vi "HP34401A.vi"(4 "error in":T14, 7 "Command":T15) -> (0 "error out":T14, 3 "Response":T12)   [LabVIEW 2018]
uses:
  MOKO_LabViewLibrary/MokoLowLevel/MokoLowLovelControl/MLLC_Command.ctl
  MOKO_LabViewLibrary/MokoLowLevel/MokoLowLovelControl/MLLC_Error.ctl
  MOKO_LabViewLibrary/MokoLowLevel/MokoLowLovelControl/MLLC_Mode.ctl
  MOKO_LabViewLibrary/MokoLowLevel/MokoLowLovelControl/MLLC_Response.ctl
  MOKO_LabViewLibrary/MokoLowLevel/MokoLowLovelControl/MLLC_DriverName.ctl
  MOKO_LabViewLibrary/MokoLowLevel/MokoLowLovelControl/MLLC_Request.ctl
  MOKO_LabViewLibrary/MokoLowLevel/MokoLowLovelControl/MLLC_ErrorCode.ctl
  MOKO_LabViewLibrary/MokoLowLevel/MokoLowLovelControl/MLLC_ResponseInit.ctl
  MOKO_LabViewLibrary/MokoLowLevel/MokoLowLovelControl/MLLC_ConnectCluster.ctl
  MOKO_LabViewLibrary/MokoLowLevel/MokoLowLovelControl/MLLC_InterfaceType.ctl
  MOKO_LabViewLibrary/MokoLowLevel/MokoLowLovelControl/MLLC_OpenedSession.ctl
  MOKO_LabViewLibrary/MokoLowLevel/MokoLowLovelControl/MLLC_InterfaceSettings.ctl
  MOKO_LabViewLibrary/MokoLowLevel/MokoLowLovelControl/MLLC_InterfaceKind.ctl
  data/HP34401A_Functions.ctl
  MOKO_LabViewLibrary/MokoLowLevel/MokoLowLovelControl/MLLC_Delay.ctl
panel:
  in  "Settings":T8={"Saved Data"=variant, "Data"={"Connect"={"InterfaceType"=enum."VISA", "OpenedSession"="", "InterfaceSettings"={"Interface"=enum."RS232", "EOS 4 read"=enum."LF (\\n)", "EOS 4 write"=enum."CR+LF (\\r\\n)", "TMO, ms"=5000, "Sett"=variant(cluster{"Baud Rate":u32, "Data Bits":u16, "Parity":u16, "Stop Bits":u16, "Flow Control":u16, "Eho":bool} {"Baud Rate"=75, "Data Bits"=0, "Parity"=0, "Stop Bits"=0, "Flow Control"=0, "Eho"=FALSE})}}, "Channel"=1, "Func"=enum."VDC"}}
  in  "Response Init array":T9="HEWLETT-PACKARD,34401A,0,10-5-2"
  in  "Error Code":T6=5475
  in  "Request":T10="*idn?"
  in  "Driver Name":T11="HP34401A_GERMAN"
  in  "Mode":T13=enum."Check"
  # "HP34401A"
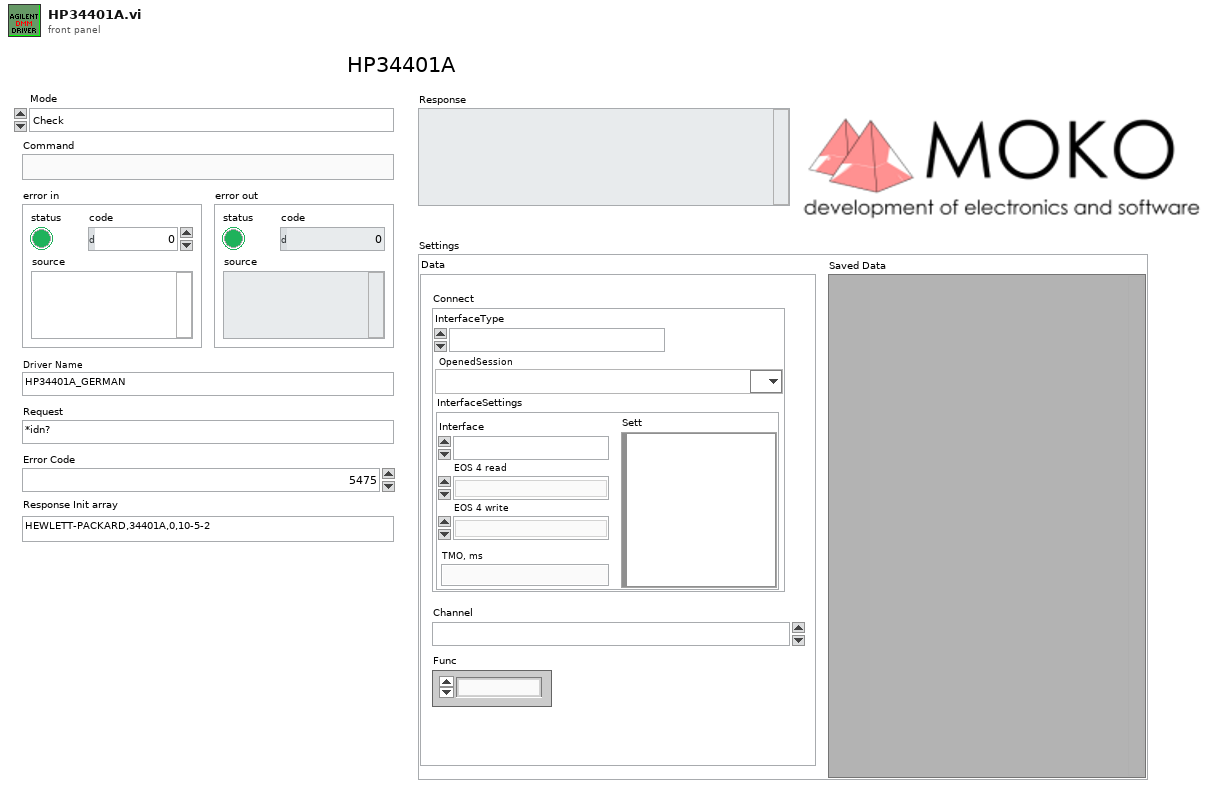
[diagram p1: front panel]
types:
  T1 = typedef "MLLC_ConnectCluster.ctl" = cluster{"InterfaceType":T2, "OpenedSession":T3, "InterfaceSettings":T4}
  T2 = typedef "MLLC_InterfaceType.ctl" = enum16{"VISA", "Prologix USB-GPIB"}
  T3 = typedef "MLLC_OpenedSession.ctl" = refnum<visa-resource-name>
  T4 = typedef "MLLC_InterfaceSettings.ctl" = cluster{"Interface":T5, "EOS 4 read":enum16{"Default (=EOS 4 write)", "CR (\\r)", "LF (\\n)", "None"}, "EOS 4 write":enum16{"CR+LF (\\r\\n)", "CR (\\r)", "LF (\\n)", "None"}, "TMO, ms":i32, "Sett":variant}
  T5 = typedef "MLLC_InterfaceKind.ctl" = enum16{"RS232", "GPIB", "USB", "Ethernet", "another"}
  T6 = typedef "MLLC_ErrorCode.ctl" = u32
  T7 = typedef "HP34401A_Functions.ctl" = enum16{"VDC", "VAC", "IDC", "IAC", "F", "R2", "R4", "CAP"}
  T8 = cluster{"Saved Data":variant, "Data":cluster{"Connect":T1, "Channel":T6, "Func":T7}}
  T9 = typedef "MLLC_ResponseInit.ctl" = string
  T10 = typedef "MLLC_Request.ctl" = string
  T11 = typedef "MLLC_DriverName.ctl" = string
  T12 = typedef "MLLC_Response.ctl" = string
  T13 = typedef "MLLC_Mode.ctl" = enum16{"get", "set", "close", "Init", "Check"}
  T14 = typedef "MLLC_Error.ctl" = errorcluster
  T15 = typedef "MLLC_Command.ctl" = string
  T16 = typedef "MLLC_Delay.ctl" = dbl
  T17 = typedef "MLLC_ResponseInitArray.ctl" = T9[]
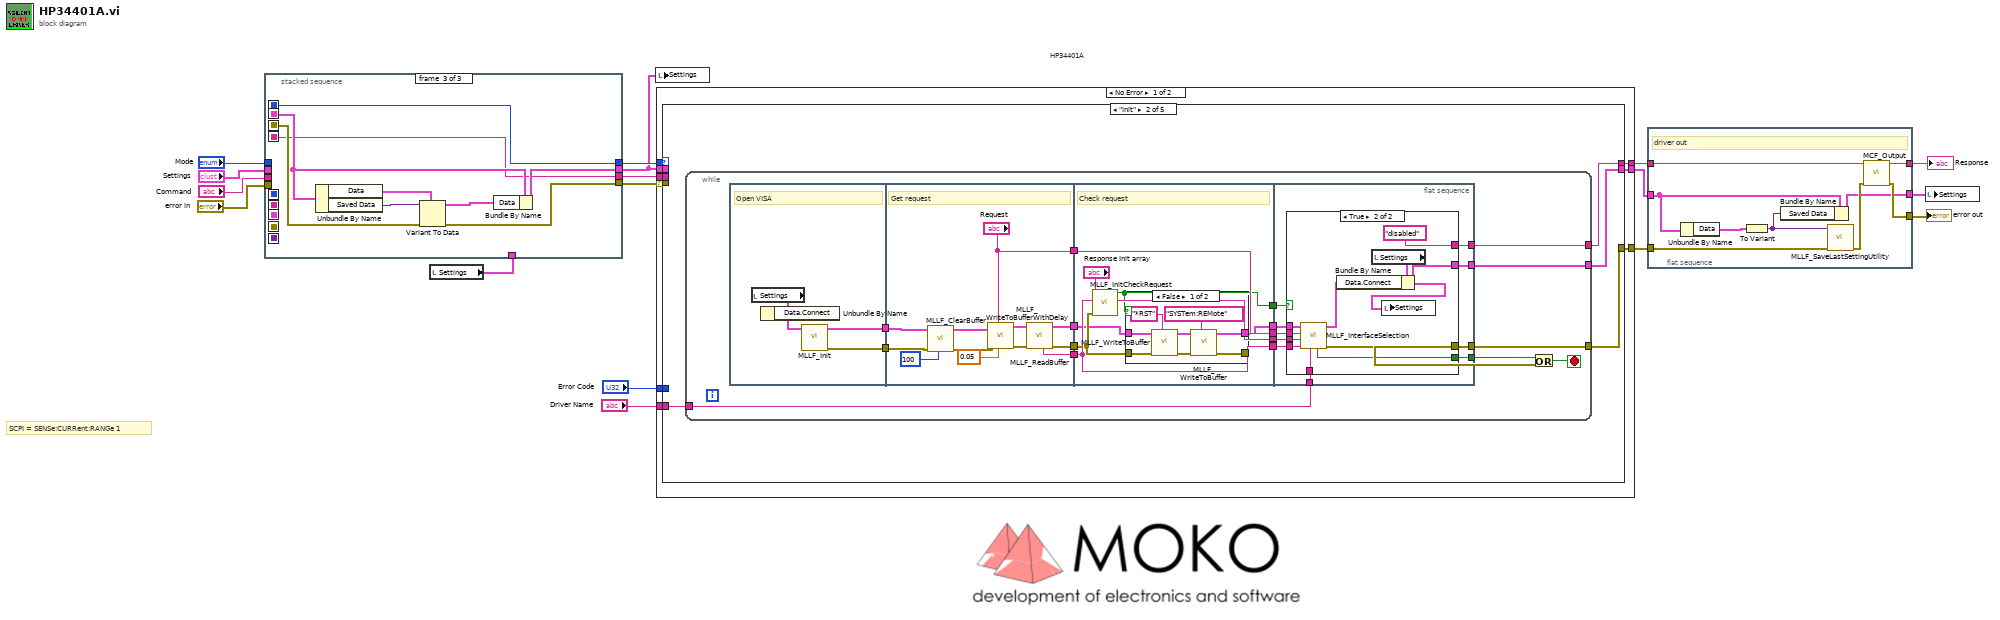
[diagram p0: block diagram]
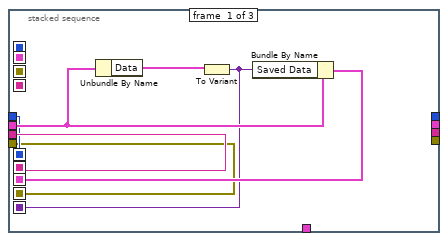
[diagram p2: hidden frame]
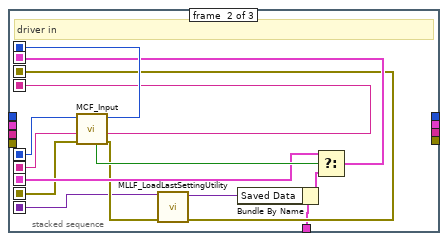
[diagram p3: hidden frame]
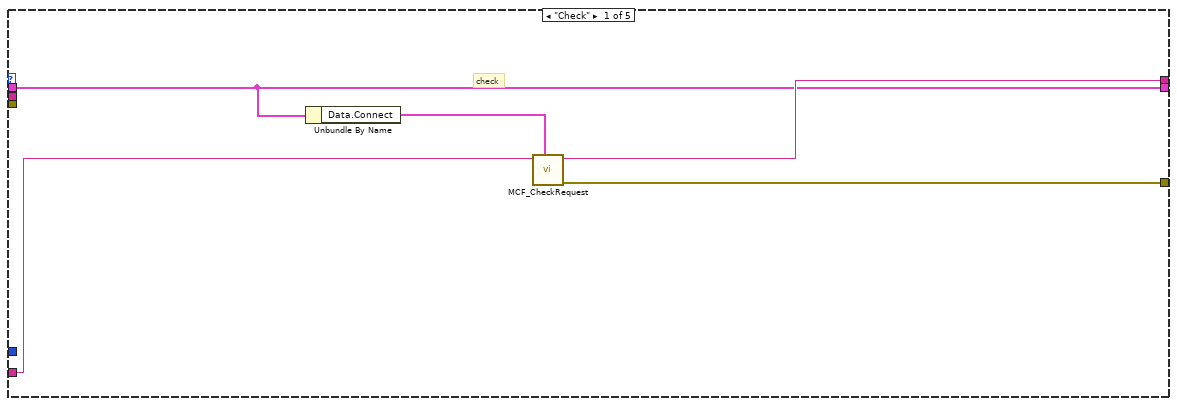
[diagram p4: hidden frame]
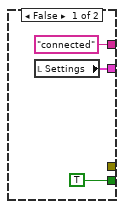
[diagram p6: hidden frame]
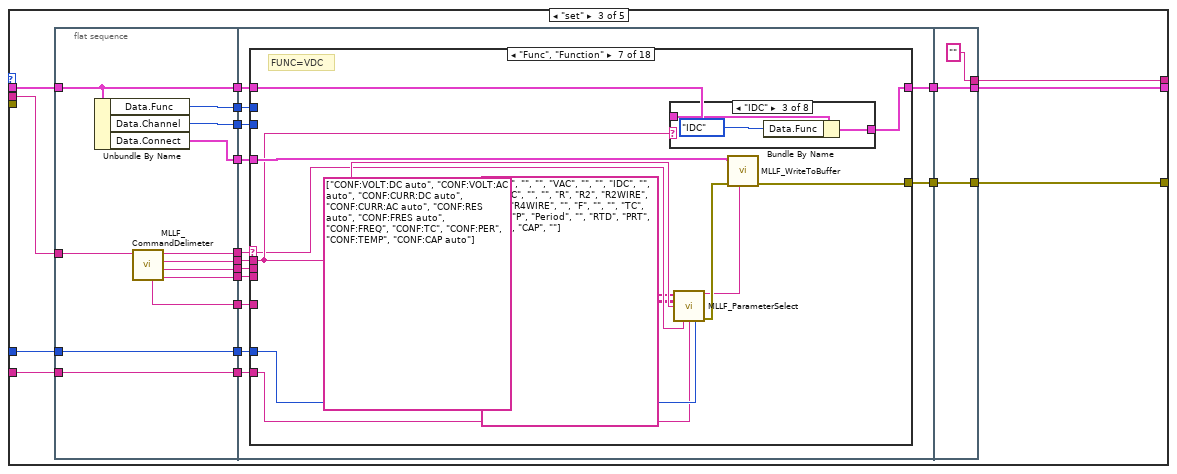
[diagram p7: hidden frame]
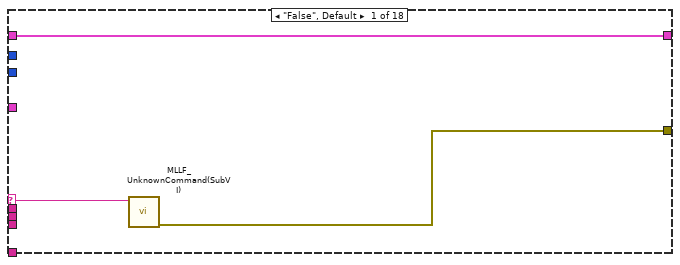
[diagram p8: hidden frame]
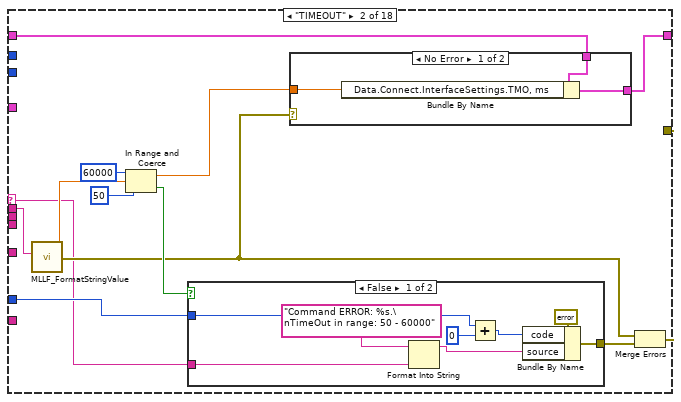
[diagram p9: hidden frame]
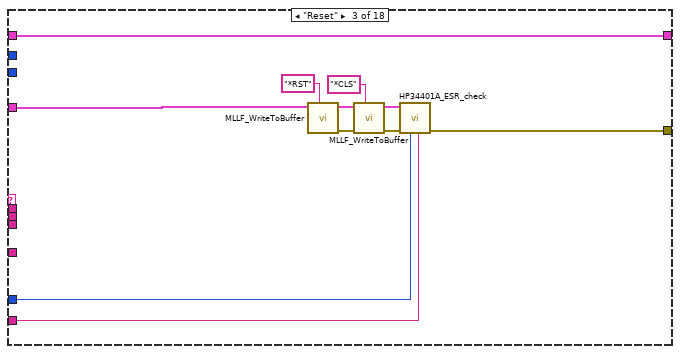
[diagram p12: hidden frame]
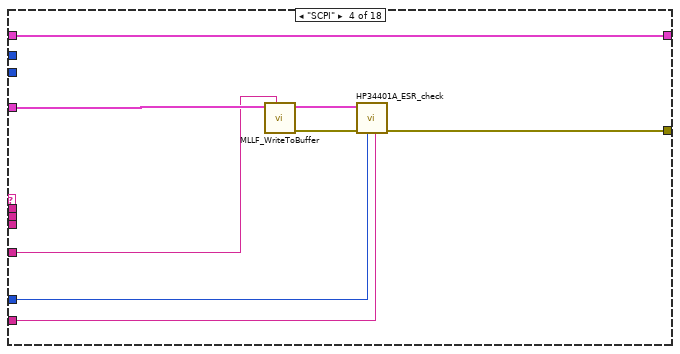
[diagram p13: hidden frame]
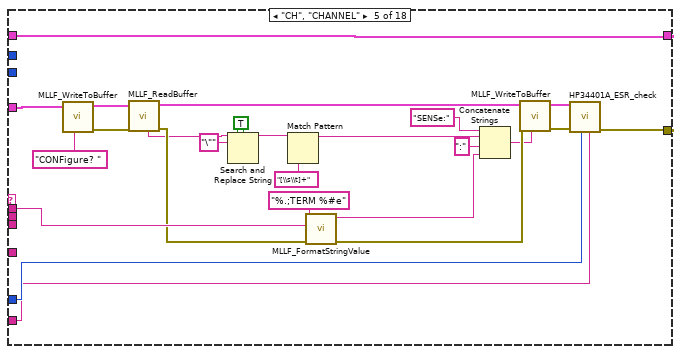
[diagram p14: hidden frame]
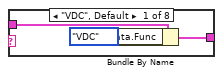
[diagram p16: hidden frame]
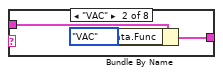
[diagram p17: hidden frame]
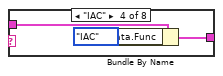
[diagram p18: hidden frame]
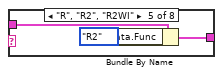
[diagram p19: hidden frame]
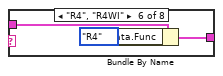
[diagram p20: hidden frame]
diagram:
  # "SCPI = SENSe:CURRent:RANGe 1"
  # "HP34401A"
  n1 = local read "Settings"() -> (w8:T8)
  n2 = stacked-sequence {
    seq-local: [w20 _ _] -> [_ w36 _]
    seq-local: [w19 _ _] -> [_ w37 _]
    seq-local: [w22 _ _] -> [_ w32 _]
    seq-local: [w18 _ _] -> [_ w31 _]
    seq-local: [w21 _ _] -> [_ w27 _]
    seq-local: [_ w28 _] -> [_ _ w44]
    seq-local: [_ w38 _] -> [_ _ w41]
    seq-local: [_ w35 _] -> [_ _ w40]
    seq-local: [_ w34 _] -> [_ _ w45]
    tunnel: "Command" -> [w20 _ _]
    tunnel: "Mode" -> [w19 _ _]
    tunnel: "error in" -> [w18 _ _]
    tunnel: "Settings" -> [w23 _ _]
    tunnel: w8 -> [_ w26 _]
    tunnel: [_ _ w40] -> w10
    tunnel: [_ _ w43] -> w1
    tunnel: [_ _ w42] -> w9
    tunnel: [_ _ w41] -> w11
    frame #0 {
      n3 = Unbundle By Name(w23) -> ("Data"=w24:cluster{"Connect":T1, "Channel":T6, "Func":T7})
      n4 = To Variant(anything=w24) -> (Variant=w21:variant)
      n5 = Bundle By Name(cluster=w23, "Saved Data"=w21) -> (w22:T8)
    }
    frame #1 {
      # "driver in"
      n6 = call "MCF_Input.vi"("Error In"=w31, "Command in"=w36, "Mode in"=w37) -> ("Error Out"=w30:errorcluster, "Command out"=w35:string, "Mode out"=w38:T13, "Boolean"=w33:bool)  [unwired: 5 in]
      n7 = call "MLLF_LoadLastSettingUtility.vi"("Error In"=w30, "Save data in"=w27) -> ("Error Out"=w28:errorcluster, "Save data out"=w25:variant)  [unwired: 8 in]
      n8 = Bundle By Name(cluster=w26, "Saved Data"=w25) -> (w29:T8)
      n9 = Select(t=w32, s=w33, f=w29) -> (s? t:f=w34:T8)
    }
    frame #2 {
      n10 = Unbundle By Name(w45) -> ("Data"=w46:cluster{"Connect":T1, "Channel":T6, "Func":T7}, "Saved Data"=w39:variant)
      n11 = Variant To Data(error in=w44, type=w46, Variant=w39) -> (data=w47:cluster{"Connect":T1, "Channel":T6, "Func":T7}, error out=w42:errorcluster)
      n12 = Bundle By Name(cluster=w45, "Data"=w47) -> (w43:T8)
    }
  }
  n13 = local write "Settings"(w1) -> ()
  n14 = case shown="No Error" w9 {
    selector: w9 -> [w53 w658]
    tunnel: [w54 w658] -> w5
    tunnel: w11 -> [w56 _]
    tunnel: [w55 "An error occurred in the driver input module." ("String")] -> w7
    tunnel: w10 -> [w48 _]
    tunnel: w1 -> [w49 w657]
    tunnel: "Error Code" -> [w52 _]
    tunnel: "Driver Name" -> [w51 _]
    tunnel: [w50 w657] -> w6
    frame No Error {
      n15 = case shown="\"Init\"" w56 {
        tunnel: [w60 w65 w153 w572 "" ("String")] -> w55
        tunnel: [w61 w63 w156 w573 w654] -> w54
        tunnel: w53 -> [_ _ _ w587 _]
        tunnel: w52 -> [_ _ w159 w589 _]
        tunnel: w51 -> [w59 w62 w157 w588 _]
        tunnel: [w57 w64 w158 w590 w653] -> w50
        tunnel: w49 -> [w57 _ w142 w578 w653]
        tunnel: w48 -> [_ _ w141 w577 _]
        frame "Check" {
          # "check"
          n16 = Unbundle By Name(w57) -> ("Data.Connect"=w58:T1)
          n17 = call "MCF_CheckRequest.vi"("Permanent data.Connect"=w58, "Driver Name"=w59) -> ("Error Out"=w61:errorcluster, "Output String"=w60:string)  [unwired: 8 in]
        }
        frame "Init" {
          n18 = while {
            tunnel: [w71] -> w63
            tunnel: [w70] -> w65
            tunnel: [w69] -> w64
            tunnel: w62 -> [w73]
            stop <- w82 stop-if-true
            n19 = flat-sequence {
              tunnel: [w86] -> w81
              tunnel: [w85] -> w80
              tunnel: w81 -> [w90]
              tunnel: w80 -> [w91]
              tunnel: [w96] -> w79
              tunnel: [w95] -> w78
              tunnel: [w94] -> w77
              tunnel: ["Request"] -> w67
              tunnel: w79 -> [w101]
              tunnel: w78 -> [w100]
              tunnel: w77 -> [w106]
              tunnel: [w99] -> w76
              tunnel: [w106] -> w75
              tunnel: [w102] -> w74
              tunnel: [w104] -> w68
              tunnel: w67 -> [w103]
              tunnel: [w103] -> w66
              tunnel: w76 -> [w124]
              tunnel: w75 -> [w123]
              tunnel: w74 -> [w125]
              tunnel: w73 -> [w122]
              tunnel: [w121] -> w72
              tunnel: [w120] -> w71
              tunnel: [w119] -> w70
              tunnel: [w118] -> w69
              tunnel: w68 -> [w117]
              tunnel: w66 -> [w116]
              frame #0 {
                # "Open VISA"
                n20 = local read "Settings"() -> (w84:T8)
                n21 = Unbundle By Name(w84) -> ("Data.Connect"=w83:T1)
                n22 = call "MLLF_Init.vi"("DriverConnect in"=w83) -> ("Error Out"=w86:errorcluster, "DriverConnect out"=w85:T1)  [unwired: 7 in]
              }
              frame #1 {
                # "Get request"
                n23 = call "MLLF_ClearBuffer.vi"("Timeout(default = 300 ms)"=u32 100, "Error In"=w90, "DriverConnect in"=w91) -> ("Error Out"=w88:errorcluster, "DriverConnect out"=w89:T1)  [unwired: 5 in, 1 out]
                n24 = call "MLLF_WriteToBufferWithDelay.vi"("Delay Time ( 0,05 s)"=T16 0.05, "Command"="Request", "Error In"=w88, "DriverConnect in"=w89) -> ("Error Out"=w97:errorcluster, "DriverConnect out"=w98:T1)  [unwired: 6 in]
                n25 = call "MLLF_ReadBuffer.vi"("Error In"=w97, "DriverConnect in"=w98) -> ("Error Out"=w96:errorcluster, "DriverConnect out"=w95:T1, "String"=w94:string)  [unwired: 6 in]
              }
              frame #2 {
                # "Check request"
                n26 = call "MLLF_InitCheckRequest.vi"("error in (no error)"=w101, "Answer"=w106, "Response Init"="Response Init array") -> ("ResponseInit out"=w104:string, "Design"=w102:bool)  [unwired: 5 in, 2 out]
                n27 = case shown="False" w102 {
                  tunnel: w101 -> [w110 _]
                  tunnel: w100 -> [w109 w115]
                  tunnel: [w108 w115] -> w99
                  tunnel: [w107 _] -> _
                  frame False {
                    n28 = call "MLLF_WriteToBuffer.vi"("String"="*RST", "error in"=w110, "DriverConnect in"=w109) -> ("error out"=w111:T14, "DriverConnect out"=w112:T1)  [unwired: 5 in]
                    n29 = call "MLLF_WriteToBuffer.vi"("String"="SYSTem:REMote", "error in"=w111, "DriverConnect in"=w112) -> ("error out"=w107:T14, "DriverConnect out"=w108:T1)  [unwired: 5 in]
                  }
                  frame True {
                  }
                }
              }
              frame #3 {
                n30 = case shown="True" w125 {
                  tunnel: w124 -> [_ w138]
                  tunnel: [TRUE w133] -> w121
                  tunnel: [_ w136] -> w120
                  tunnel: ["connected" "disabled"] -> w119
                  tunnel: [w126 w134] -> w118
                  tunnel: w123 -> [_ w131]
                  tunnel: w122 -> [_ w132]
                  tunnel: w117 -> [_ w130]
                  tunnel: w116 -> [_ w129]
                  frame False {
                    n31 = local read "Settings"() -> (w126:T8)
                  }
                  frame True {
                    n32 = call "MLLF_InterfaceSelection.vi"("Driver Name"=w132, "Answer:"=w131, "Response"=w130, "Request"=w129, "DriverConnect in"=w138) -> ("error out"=w136:T14, "DriverConnect out"=w137:T1, "stop init?"=w133:bool)  [unwired: 2 in, 2 out]
                    n33 = local read "Settings"() -> (w139:T8)
                    n34 = Bundle By Name(cluster=w139, "Data.Connect"=w137) -> (w134:T8)
                    n35 = local write "Settings"(w134) -> ()
                  }
                }
              }
            }
            n36 = Or(x=w72, y=w71) -> (x .or. y?=w82:bool)
          }
        }
        frame "set" {
          n37 = flat-sequence {
            tunnel: w157 -> [w170]
            tunnel: w142 -> [w161]
            tunnel: w159 -> [w171]
            tunnel: [w171] -> w152
            tunnel: [w161] -> w151
            tunnel: [w170] -> w150
            tunnel: [w167] -> w149
            tunnel: [w168] -> w148
            tunnel: [w169] -> w147
            tunnel: [w162] -> w146
            tunnel: [w163] -> w145
            tunnel: [w164] -> w144
            tunnel: [w165] -> w143
            tunnel: w141 -> [w166]
            tunnel: [w160] -> w140
            tunnel: [w182] -> w155
            tunnel: [w175] -> w154
            tunnel: w152 -> [w184]
            tunnel: w151 -> [w183]
            tunnel: w150 -> [w181]
            tunnel: w149 -> [w180]
            tunnel: w148 -> [w179]
            tunnel: w147 -> [w178]
            tunnel: w146 -> [w177]
            tunnel: w145 -> [w176]
            tunnel: w144 -> [w174]
            tunnel: w143 -> [w173]
            tunnel: w140 -> [w172]
            tunnel: [w570] -> w156
            tunnel: [w571] -> w158
            tunnel: w155 -> [w571]
            tunnel: w154 -> [w570]
            tunnel: ["" ("String")] -> w153
            frame #0 {
              n38 = Unbundle By Name(w161) -> ("Data.Func"=w169:T7, "Data.Channel"=w168:T6, "Data.Connect"=w167:T1)
              n39 = call "MLLF_CommandDelimeter.vi"("command with param"=w166) -> ("param 3"=w165:string, "param 2"=w164:string, "param 1"=w163:string, "command"=w162:string, "Spit delimetre"=w160:string)  [unwired: 6 in]
            }
            frame #1 {
              n40 = case shown="\"Func\", \"Function\"" w177 {
                selector: w177 -> [w186 w189 _ _ _ _ w263 _ _ _ _ _ _ w484 w491 w517 w543 w556]
                tunnel: w176 -> [_ w188 _ _ w251 _ w264 w311 _ w344 w359 w406 w442 w485 w492 w518 w544 w557]
                tunnel: [w185 w194 w214 w228 w253 _ w258 w294 _ w348 w377 w410 w446 w489 w513 w539 w552 w563] -> w175
                tunnel: w184 -> [_ w195 w216 w230 w256 _ w269 _ _ w347 w376 w409 w445 w486 w496 w522 w548 w565]
                tunnel: w183 -> [w187 w199 w223 w231 w252 w257 w266 w313 w325 w349 w378 w411 w447 w490 w514 w540 w553 w568]
                tunnel: [w187 w200 w223 w231 w252 w257 w265 w313 w325 w349 w378 w411 w447 w490 w514 w540 w553 w568] -> w182
                tunnel: w180 -> [_ _ w213 w227 w254 _ w267 w312 _ w345 w374 w407 w443 w488 w512 w538 w546 w561]
                tunnel: w181 -> [_ _ w215 w229 w255 _ w268 _ _ w346 w375 w408 w444 w487 w497 w523 w549 w564]
                tunnel: w179 -> [_ _ _ _ _ _ _ _ _ _ _ _ _ _ _ _ _ _]
                tunnel: w178 -> [_ _ _ _ _ _ _ _ _ _ _ _ _ _ _ _ _ _]
                tunnel: w174 -> [_ _ _ _ _ _ _ _ _ _ _ _ _ _ _ _ _ _]
                tunnel: w173 -> [_ _ _ _ _ _ _ _ _ _ _ _ _ _ _ _ _ _]
                tunnel: w172 -> [_ _ _ w224 _ _ _ _ _ _ _ _ _ _ _ _ _ _]
                frame "False", Default {
                  n41 = call "MLLF_UnknownCommand(SubVI).vi"("Unknown command"=w186) -> ("error out"=w185:errorcluster)  [unwired: 10 in]
                }
                frame "TIMEOUT" {
                  n42 = call "MLLF_FormatStringValue.vi"("String Value"=w188) -> ("error out"=w190:T14, "number"=w191:dbl)  [unwired: 8 in, 1 out]
                  n43 = In Range and Coerce(upper limit=60000, x=w191, lower limit=50) -> (coerced(x)=w196:dbl, In Range?=w192:bool)
                  n44 = case shown="False" w192 {
                    tunnel: [w207 _] -> w193
                    tunnel: w195 -> [w206 _]
                    tunnel: w189 -> [w205 _]
                    frame False {
                      n45 = Format Into String(format string="Command ERROR: %s.\nTimeOut in range: 50 - 60000", w205) -> (resulting string=w209:string)  [unwired: 2 in, 1 out]
                      n46 = Add(x=w206, y=0) -> (x+y=w210:T6)
                      n47 = Bundle By Name(cluster=errorcluster {"status"=TRUE, "code"=0, "source"=""} ("error out"), "code"=w210, "source"=w209) -> (w207:errorcluster)
                    }
                    frame True {
                    }
                  }
                  n48 = case shown="No Error" w190 {
                    tunnel: [w203 w204] -> w200
                    tunnel: w199 -> [w202 w204]
                    tunnel: w196 -> [w201 _]
                    frame No Error {
                      n49 = Bundle By Name(cluster=w202, "Data.Connect.InterfaceSettings.TMO, ms"=w201) -> (w203:T8)
                    }
                    frame Error {
                    }
                  }
                  n50 = Merge Errors(w190, w193) -> (w194:errorcluster)
                }
                frame "Reset" {
                  n51 = call "MLLF_WriteToBuffer.vi"("String"="*RST", "DriverConnect in"=w213) -> ("error out"=w221:T14, "DriverConnect out"=w222:T1)  [unwired: 6 in]
                  n52 = call "MLLF_WriteToBuffer.vi"("String"="*CLS" ("write buffer"), "error in"=w221, "DriverConnect in"=w222) -> ("error out"=w218:T14, "DriverConnect out"=w217:T1)  [unwired: 5 in]
                  n53 = call "HP34401A_ESR_check.vi"("Driver Name"=w215, "Error Code"=w216, "error in"=w218, "DriverConnect in"=w217) -> ("error out"=w214:T14)  [unwired: 6 in, 1 out]
                }
                frame "SCPI" {
                  n54 = call "MLLF_WriteToBuffer.vi"("String"=w224, "DriverConnect in"=w227) -> ("error out"=w225:T14, "DriverConnect out"=w226:T1)  [unwired: 6 in]
                  n55 = call "HP34401A_ESR_check.vi"("Driver Name"=w229, "Error Code"=w230, "error in"=w225, "DriverConnect in"=w226) -> ("error out"=w228:T14)  [unwired: 6 in, 1 out]
                }
                frame "CH", "CHANNEL" {
                  w236 = TRUE ("replace all? (F)")
                  n56 = call "MLLF_WriteToBuffer.vi"("String"="CONFigure? ", "DriverConnect in"=w254) -> ("error out"=w245:T14, "DriverConnect out"=w246:T1)  [unwired: 6 in]
                  n57 = call "MLLF_ReadBuffer.vi"("Error In"=w245, "DriverConnect in"=w246) -> ("Error Out"=w244:errorcluster, "DriverConnect out"=w243:T1, "String"=w238:string)  [unwired: 6 in]
                  n58 = Search and Replace String(replace all?=w236, case sensitive?=w236, input string=w238, search string="\"") -> (result string=w237:string)  [unwired: 4 in, 3 out]
                  n59 = Match Pattern(string=w237, regular expression="[\\s\\t]+") -> (before substring=w239:string)  [unwired: 1 in, 3 out]
                  n60 = call "MLLF_FormatStringValue.vi"("error in"=w244, "String Value"=w251, "Format"="%.;TERM %#e" ("format string")) -> ("error out"=w250:T14, "String Value Formated"=w241:T15)  [unwired: 6 in, 1 out]
                  n61 = Concatenate Strings("SENSe:" ("string"), w239, ":" ("string"), w241) -> (w234:string)
                  n62 = call "MLLF_WriteToBuffer.vi"("String"=w234, "error in"=w250, "DriverConnect in"=w243) -> ("error out"=w249:T14, "DriverConnect out"=w248:T1)  [unwired: 5 in]
                  n63 = call "HP34401A_ESR_check.vi"("Driver Name"=w255, "Error Code"=w256, "error in"=w249, "DriverConnect in"=w248) -> ("error out"=w253:T14)  [unwired: 6 in, 1 out]
                }
                frame "<----MAIN FUNCTIONS---->" {
                }
                frame "Func", "Function" {
                  # "FUNC=VDC"
                  n64 = case shown="\"IDC\"" w264 {
                    tunnel: w266 -> [w272 w275 w278 w281 w284 w287 w290 w293]
                    tunnel: [w271 w274 w277 w280 w283 w286 w289 w292] -> w265
                    frame "VDC", Default {
                      n65 = Bundle By Name(cluster=w272, "Data.Func"=HP34401A_Functions."VDC" ("Func")) -> (w271:T8)
                    }
                    frame "VAC" {
                      n66 = Bundle By Name(cluster=w275, "Data.Func"=HP34401A_Functions."VAC" ("Func")) -> (w274:T8)
                    }
                    frame "IDC" {
                      n67 = Bundle By Name(cluster=w278, "Data.Func"=HP34401A_Functions."IDC" ("Func")) -> (w277:T8)
                    }
                    frame "IAC" {
                      n68 = Bundle By Name(cluster=w281, "Data.Func"=HP34401A_Functions."IAC" ("Func")) -> (w280:T8)
                    }
                    frame "R", "R2", "R2WI" {
                      n69 = Bundle By Name(cluster=w284, "Data.Func"=HP34401A_Functions."R2" ("Func")) -> (w283:T8)
                    }
                    frame "R4", "R4WI" {
                      n70 = Bundle By Name(cluster=w287, "Data.Func"=HP34401A_Functions."R4" ("Func")) -> (w286:T8)
                    }
                    frame "F" {
                      n71 = Bundle By Name(cluster=w290, "Data.Func"=HP34401A_Functions."F" ("Func")) -> (w289:T8)
                    }
                    frame "C", "CAP" {
                      n72 = Bundle By Name(cluster=w293, "Data.Func"=HP34401A_Functions."CAP" ("Func")) -> (w292:T8)
                    }
                  }
                  n73 = call "MLLF_ParameterSelect.vi"("Command to equipment"=string[] ["CONF:VOLT:DC auto", "CONF:VOLT:AC auto", "CONF:CURR:DC auto", "CONF:CURR:AC auto", "CONF:RES auto", "CONF:FRES auto", "CONF:FREQ", "CONF:TC", "CONF:PER", "CONF:TEMP", "CONF:CAP auto"] ("Names"), "Names"=string[][] [["VDC", "", ""], ["VAC", "", ""], ["IDC", "", ""], ["IAC", "", ""], ["R", "R2", "R2WIRE"], ["R4", "R4WIRE", ""], ["F", "", ""], ["TC", "", ""], ["P", "Period", ""], ["RTD", "PRT", ""], ["C", "CAP", ""]], "Input"=w264, "Command"=w263, "Driver Name"=w268, "Error Code"=w269) -> ("Choice"=w259:string, "Error Out"=w260:errorcluster)  [unwired: 8 in]
                  n74 = call "MLLF_WriteToBuffer.vi"("String"=w259, "error in"=w260, "DriverConnect in"=w267) -> ("error out"=w258:T14)  [unwired: 5 in, 1 out]
                }
                frame "Range" {
                  w299 = TRUE ("replace all? (F)")
                  n75 = call "MLLF_WriteToBuffer.vi"("String"="CONFigure? ", "DriverConnect in"=w312) -> ("error out"=w307:T14, "DriverConnect out"=w308:T1)  [unwired: 6 in]
                  n76 = call "MLLF_ReadBuffer.vi"("Error In"=w307, "DriverConnect in"=w308) -> ("Error Out"=w296:errorcluster, "DriverConnect out"=w306:T1, "String"=w301:string)  [unwired: 6 in]
                  n77 = Search and Replace String(replace all?=w299, case sensitive?=w299, input string=w301, search string="\"") -> (result string=w300:string)  [unwired: 4 in, 3 out]
                  n78 = case shown="\"MIN\"" w311 {
                    selector: w311 -> [w315 _ _ _]
                    tunnel: [w318 w319 w321 w323] -> w310
                    tunnel: [w317 "RANG:AUTO ON" ("String") "RANG MIN" ("String") "RANG MAX" ("String")] -> w304
                    tunnel: w296 -> [w314 w319 w321 w323]
                    frame "False", Default {
                      n79 = call "MLLF_FormatStringValue.vi"("error in"=w314, "String Value"=w315, "Format"="RANG %#e" ("format string")) -> ("error out"=w318:T14, "String Value Formated"=w317:T15)  [unwired: 6 in, 1 out]
                    }
                    frame "Auto" {
                    }
                    frame "MIN" {
                    }
                    frame "MAX" {
                    }
                  }
                  n80 = Match Pattern(string=w300, regular expression="[\\s\\t]+") -> (before substring=w302:string)  [unwired: 1 in, 3 out]
                  n81 = Concatenate Strings("SENSe:" ("string"), w302, ":" ("string"), w304) -> (w297:string)
                  n82 = call "MLLF_WriteToBuffer.vi"("String"=w297, "error in"=w310, "DriverConnect in"=w306) -> ("error out"=w294:T14)  [unwired: 5 in, 1 out]
                }
                frame "---------ADDITIONAL---------" {
                }
                frame "Res", "Resolution" {
                  w329 = TRUE ("replace all? (F)")
                  n83 = call "MLLF_WriteToBuffer.vi"("String"="CONFigure? ", "DriverConnect in"=w345) -> ("error out"=w338:T14, "DriverConnect out"=w339:T1)  [unwired: 6 in]
                  n84 = call "MLLF_ReadBuffer.vi"("Error In"=w338, "DriverConnect in"=w339) -> ("Error Out"=w337:errorcluster, "DriverConnect out"=w336:T1, "String"=w331:string)  [unwired: 6 in]
                  n85 = Search and Replace String(replace all?=w329, case sensitive?=w329, input string=w331, search string="\"") -> (result string=w330:string)  [unwired: 4 in, 3 out]
                  n86 = case shown="\"MIN\"" w344 {
                    selector: w344 -> [w351 _ _]
                    tunnel: [w354 w355 w357] -> w343
                    tunnel: [w353 "RES MAX" ("String") "RES MIN" ("String")] -> w334
                    tunnel: w337 -> [w350 w355 w357]
                    frame "False", Default {
                      n87 = call "MLLF_FormatStringValue.vi"("error in"=w350, "String Value"=w351, "Format"="RES %#e" ("format string")) -> ("error out"=w354:T14, "String Value Formated"=w353:T15)  [unwired: 6 in, 1 out]
                    }
                    frame "MAX" {
                    }
                    frame "MIN" {
                    }
                  }
                  n88 = Match Pattern(string=w330, regular expression="[\\s\\t]+") -> (before substring=w332:string)  [unwired: 1 in, 3 out]
                  n89 = Concatenate Strings("SENSe:" ("string"), w332, ":" ("string"), w334) -> (w327:string)
                  n90 = call "MLLF_WriteToBuffer.vi"("String"=w327, "error in"=w343, "DriverConnect in"=w336) -> ("error out"=w342:T14, "DriverConnect out"=w341:T1)  [unwired: 5 in]
                  n91 = call "HP34401A_ESR_check.vi"("Driver Name"=w346, "Error Code"=w347, "error in"=w342, "DriverConnect in"=w341) -> ("error out"=w348:T14)  [unwired: 6 in, 1 out]
                }
                frame "Aper", "Aperture", "MeasTime" {
                  w362 = TRUE ("replace all? (F)")
                  n92 = call "MLLF_WriteToBuffer.vi"("String"="CONFigure? ", "DriverConnect in"=w374) -> ("error out"=w371:T14, "DriverConnect out"=w372:T1)  [unwired: 6 in]
                  n93 = call "MLLF_ReadBuffer.vi"("Error In"=w371, "DriverConnect in"=w372) -> ("Error Out"=w370:errorcluster, "DriverConnect out"=w369:T1, "String"=w364:string)  [unwired: 6 in]
                  n94 = Search and Replace String(replace all?=w362, case sensitive?=w362, input string=w364, search string="\"") -> (result string=w363:string)  [unwired: 4 in, 3 out]
                  n95 = case shown="\"OFF\"" w359 {
                    selector: w359 -> [w383 _]
                    tunnel: [w386 w387] -> w381
                    tunnel: [w385 "APER:ENAB OFF" ("String")] -> w367
                    tunnel: w370 -> [w382 w387]
                    frame "False", Default {
                      n96 = call "MLLF_FormatStringValue.vi"("error in"=w382, "String Value"=w383, "Format"="APER %#e" ("format string")) -> ("error out"=w386:T14, "String Value Formated"=w385:T15)  [unwired: 6 in, 1 out]
                    }
                    frame "OFF" {
                    }
                  }
                  n97 = Match Pattern(string=w363, regular expression="[\\s\\t]+") -> (before substring=w365:string)  [unwired: 1 in, 3 out]
                  n98 = Concatenate Strings(w365, ":" ("string"), w367) -> (w360:string)
                  n99 = call "MLLF_WriteToBuffer.vi"("String"=w360, "error in"=w381, "DriverConnect in"=w369) -> ("error out"=w380:T14, "DriverConnect out"=w379:T1)  [unwired: 5 in]
                  n100 = call "HP34401A_ESR_check.vi"("Driver Name"=w375, "Error Code"=w376, "error in"=w380, "DriverConnect in"=w379) -> ("error out"=w377:T14)  [unwired: 6 in, 1 out]
                }
                frame "IntegrationTime", "IntTime", "NPLC" {
                  w392 = TRUE ("replace all? (F)")
                  n101 = call "MLLF_WriteToBuffer.vi"("String"="CONFigure? ", "DriverConnect in"=w407) -> ("error out"=w400:T14, "DriverConnect out"=w401:T1)  [unwired: 6 in]
                  n102 = call "MLLF_ReadBuffer.vi"("Error In"=w400, "DriverConnect in"=w401) -> ("DriverConnect out"=w399:T1, "String"=w394:string)  [unwired: 6 in, 1 out]
                  n103 = Search and Replace String(replace all?=w392, case sensitive?=w392, input string=w394, search string="\"") -> (result string=w393:string)  [unwired: 4 in, 3 out]
                  n104 = case shown="\"MIN\"" w406 {
                    tunnel: [w415 w419 w423] -> w405
                    tunnel: [w414 w418 w422] -> w397
                    tunnel: w406 -> [w412 w416 w420]
                    frame Default {
                      n105 = call "MLLF_FormatStringValue.vi"("String Value"=w412, "Format"="NPLC %#e" ("format string")) -> ("error out"=w415:T14, "String Value Formated"=w414:T15)  [unwired: 7 in, 1 out]
                    }
                    frame "MIN" {
                      n106 = call "MLLF_FormatStringValue.vi"("String Value"=w416, "Format"="NPLC MIN" ("format string")) -> ("error out"=w419:T14, "String Value Formated"=w418:T15)  [unwired: 7 in, 1 out]
                    }
                    frame "MAX" {
                      n107 = call "MLLF_FormatStringValue.vi"("String Value"=w420, "Format"="NPLC MAX" ("format string")) -> ("error out"=w423:T14, "String Value Formated"=w422:T15)  [unwired: 7 in, 1 out]
                    }
                  }
                  n108 = Match Pattern(string=w393, regular expression="[\\s\\t]+") -> (before substring=w395:string)  [unwired: 1 in, 3 out]
                  n109 = Concatenate Strings("SENSe:" ("string"), w395, ":" ("string"), w397) -> (w390:string)
                  n110 = call "MLLF_WriteToBuffer.vi"("String"=w390, "error in"=w405, "DriverConnect in"=w399) -> ("error out"=w404:T14, "DriverConnect out"=w403:T1)  [unwired: 5 in]
                  n111 = call "HP34401A_ESR_check.vi"("Driver Name"=w408, "Error Code"=w409, "error in"=w404, "DriverConnect in"=w403) -> ("error out"=w410:T14)  [unwired: 6 in, 1 out]
                }
                frame "ACBand", "ACBandwidth", "Band", "Bandwidth" {
                  w429 = TRUE ("replace all? (F)")
                  n112 = call "MLLF_WriteToBuffer.vi"("String"="CONFigure? ", "DriverConnect in"=w443) -> ("error out"=w436:T14, "DriverConnect out"=w437:T1)  [unwired: 6 in]
                  n113 = call "MLLF_ReadBuffer.vi"("Error In"=w436, "DriverConnect in"=w437) -> ("Error Out"=w435:errorcluster, "DriverConnect out"=w434:T1, "String"=w431:string)  [unwired: 6 in]
                  n114 = case shown="Default" w442 {
                    tunnel: [w452 w457 w462] -> w441
                    tunnel: w435 -> [w451 w456 w461]
                    tunnel: [w450 w455 w460] -> w432
                    tunnel: w442 -> [w448 w453 w458]
                    frame Default {
                      n115 = call "MLLF_FormatStringValue.vi"("error in"=w451, "String Value"=w448, "Format"="BAND %#f" ("format string")) -> ("error out"=w452:T14, "String Value Formated"=w450:T15)  [unwired: 6 in, 1 out]
                    }
                    frame "MAX" {
                      n116 = call "MLLF_FormatStringValue.vi"("error in"=w456, "String Value"=w453, "Format"="BAND MAX" ("format string")) -> ("error out"=w457:T14, "String Value Formated"=w455:T15)  [unwired: 6 in, 1 out]
                    }
                    frame "MIN" {
                      n117 = call "MLLF_FormatStringValue.vi"("error in"=w461, "String Value"=w458, "Format"="BAND MIN" ("format string")) -> ("error out"=w462:T14, "String Value Formated"=w460:T15)  [unwired: 6 in, 1 out]
                    }
                  }
                  n118 = Search and Replace String(replace all?=w429, case sensitive?=w429, input string=w431, search string="\"") -> (result string=w430:string)  [unwired: 4 in, 3 out]
                  n119 = Match Pattern(string=w430, regular expression="[\\s\\t]+") -> (before substring=w425:string)  [unwired: 1 in, 3 out]
                  n120 = Concatenate Strings("SENSe:" ("string"), w425, ":DET:" ("string"), w432) -> (w427:string)
                  n121 = call "MLLF_WriteToBuffer.vi"("String"=w427, "error in"=w441, "DriverConnect in"=w434) -> ("error out"=w440:T14, "DriverConnect out"=w439:T1)  [unwired: 5 in]
                  n122 = call "HP34401A_ESR_check.vi"("Driver Name"=w444, "Error Code"=w445, "error in"=w440, "DriverConnect in"=w439) -> ("error out"=w446:T14)  [unwired: 6 in, 1 out]
                }
                frame "AutoZero", "ZERO" {
                  w472 = TRUE ("replace all? (F)")
                  n123 = call "MLLF_WriteToBuffer.vi"("String"="CONFigure? ", "DriverConnect in"=w488) -> ("error out"=w479:T14, "DriverConnect out"=w480:T1)  [unwired: 6 in]
                  n124 = call "MLLF_ReadBuffer.vi"("Error In"=w479, "DriverConnect in"=w480) -> ("Error Out"=w466:errorcluster, "DriverConnect out"=w478:T1, "String"=w474:string)  [unwired: 6 in]
                  n125 = Search and Replace String(replace all?=w472, case sensitive?=w472, input string=w474, search string="\"") -> (result string=w473:string)  [unwired: 4 in, 3 out]
                  n126 = Match Pattern(string=w473, regular expression="[\\s\\t]+") -> (before substring=w475:string)  [unwired: 1 in, 3 out]
                  n127 = call "MLLF_ParameterSelect.vi"("Command to equipment"=string[] ["ZERO:AUTO OFF", "ZERO:AUTO ON", "ZERO:AUTO ONCE"] ("Names"), "Ignor case(default = true)"=TRUE, "Names"=string[][] [["OFF"], ["ON"], ["ONCE"]], "Input"=w485, "Error In"=w466, "Command"=w484, "Driver Name"=w487, "Error Code"=w486) -> ("Choice"=w465:string, "Error Out"=w467:errorcluster)  [unwired: 6 in]
                  n128 = Concatenate Strings("SENSe:" ("string"), w475, ":" ("string"), w465) -> (w470:string)
                  n129 = call "MLLF_WriteToBuffer.vi"("String"=w470, "error in"=w467, "DriverConnect in"=w478) -> ("error out"=w483:T14, "DriverConnect out"=w482:T1)  [unwired: 5 in]
                  n130 = call "HP34401A_ESR_check.vi"("Driver Name"=w487, "Error Code"=w486, "error in"=w483, "DriverConnect in"=w482) -> ("error out"=w489:T14)  [unwired: 6 in, 1 out]
                }
                frame "LOWPOWER" {
                  w502 = TRUE ("replace all? (F)")
                  n131 = call "MLLF_WriteToBuffer.vi"("String"="CONFigure? ", "DriverConnect in"=w512) -> ("error out"=w509:T14, "DriverConnect out"=w510:T1)  [unwired: 6 in]
                  n132 = call "MLLF_ReadBuffer.vi"("Error In"=w509, "DriverConnect in"=w510) -> ("Error Out"=w494:errorcluster, "DriverConnect out"=w508:T1, "String"=w504:string)  [unwired: 6 in]
                  n133 = Search and Replace String(replace all?=w502, case sensitive?=w502, input string=w504, search string="\"") -> (result string=w503:string)  [unwired: 4 in, 3 out]
                  n134 = Match Pattern(string=w503, regular expression="[\\s\\t]+") -> (before substring=w505:string)  [unwired: 1 in, 3 out]
                  n135 = call "MLLF_ParameterSelect.vi"("Command to equipment"=string[] ["POW:LIM OFF", "POW:LIM ON"] ("Names"), "Names"=string[][] [["0", "DIS", "DISABLE", "DISABLED", "OFF"], ["1", "EN", "ENABLE", "ENABLED", "ON"]], "Input"=w492, "Error In"=w494, "Command"=w491, "Driver Name"=w497, "Error Code"=w496) -> ("Choice"=w493:string, "Error Out"=w495:errorcluster)  [unwired: 7 in]
                  n136 = Concatenate Strings(w505, ":" ("string"), w493) -> (w500:string)
                  n137 = call "MLLF_WriteToBuffer.vi"("String"=w500, "error in"=w495, "DriverConnect in"=w508) -> ("error out"=w516:T14, "DriverConnect out"=w515:T1)  [unwired: 5 in]
                  n138 = call "HP34401A_ESR_check.vi"("Driver Name"=w497, "Error Code"=w496, "error in"=w516, "DriverConnect in"=w515) -> ("error out"=w513:T14)  [unwired: 6 in, 1 out]
                }
                frame "VOLTAGELIMITED" {
                  w528 = TRUE ("replace all? (F)")
                  n139 = call "MLLF_WriteToBuffer.vi"("String"="CONFigure? ", "DriverConnect in"=w538) -> ("error out"=w535:T14, "DriverConnect out"=w536:T1)  [unwired: 6 in]
                  n140 = call "MLLF_ReadBuffer.vi"("Error In"=w535, "DriverConnect in"=w536) -> ("Error Out"=w520:errorcluster, "DriverConnect out"=w534:T1, "String"=w530:string)  [unwired: 6 in]
                  n141 = Search and Replace String(replace all?=w528, case sensitive?=w528, input string=w530, search string="\"") -> (result string=w529:string)  [unwired: 4 in, 3 out]
                  n142 = Match Pattern(string=w529, regular expression="[\\s\\t]+") -> (before substring=w531:string)  [unwired: 1 in, 3 out]
                  n143 = call "MLLF_ParameterSelect.vi"("Command to equipment"=string[] ["VOLT:LIM OFF", "VOLT:LIM ON"] ("Names"), "Names"=string[][] [["0", "DIS", "DISABLE", "DISABLED", "OFF"], ["1", "EN", "ENABLE", "ENABLED", "ON"]], "Input"=w518, "Error In"=w520, "Command"=w517, "Driver Name"=w523, "Error Code"=w522) -> ("Choice"=w519:string, "Error Out"=w521:errorcluster)  [unwired: 7 in]
                  n144 = Concatenate Strings(w531, ":" ("string"), w519) -> (w526:string)
                  n145 = call "MLLF_WriteToBuffer.vi"("String"=w526, "error in"=w521, "DriverConnect in"=w534) -> ("error out"=w542:T14, "DriverConnect out"=w541:T1)  [unwired: 5 in]
                  n146 = call "HP34401A_ESR_check.vi"("Driver Name"=w523, "Error Code"=w522, "error in"=w542, "DriverConnect in"=w541) -> ("error out"=w539:T14)  [unwired: 6 in, 1 out]
                }
                frame "FILT", "FILTER" {
                  # "FILT=DIS"
                  n147 = call "MLLF_ParameterSelect.vi"("Command to equipment"=string[] ["INPut:FILTer:STATE OFF", "INPut:FILTer:STATE ON"] ("Names"), "Names"=string[][] [["0", "DIS", "DISABLE", "DISABLED", "OFF"], ["1", "EN", "ENABLE", "ENABLED", "ON"]], "Input"=w544, "Command"=w543, "Driver Name"=w549, "Error Code"=w548) -> ("Choice"=w545:string, "Error Out"=w547:errorcluster)  [unwired: 8 in]
                  n148 = call "MLLF_WriteToBuffer.vi"("String"=w545, "error in"=w547, "DriverConnect in"=w546) -> ("error out"=w555:T14, "DriverConnect out"=w554:T1)  [unwired: 5 in]
                  n149 = call "HP34401A_ESR_check.vi"("Driver Name"=w549, "Error Code"=w548, "error in"=w555, "DriverConnect in"=w554) -> ("error out"=w552:T14)  [unwired: 6 in, 1 out]
                }
                frame "SND", "Sound" {
                  # "sound"
                  # "sound=off"
                  n150 = call "MLLF_ParameterSelect.vi"("Command to equipment"=string[] ["SYST:BEEP:STAT OFF", "SYST:BEEP:STAT ON", "SYST:BEEP"] ("Names"), "Names"=string[][] [["0", "DIS", "DISABLED", "DISABLE", "OFF"], ["1", "EN", "ENABLE", "ENABLED", "ON"], [" ", "", "", "", ""]], "Input"=w557, "Command"=w556, "Driver Name"=w564, "Error Code"=w565) -> ("Choice"=w560:string, "Error Out"=w562:errorcluster)  [unwired: 8 in]
                  n151 = call "MLLF_WriteToBuffer.vi"("String"=w560, "error in"=w562, "DriverConnect in"=w561) -> ("error out"=w567:T14, "DriverConnect out"=w566:T1)  [unwired: 5 in]
                  n152 = call "HP34401A_ESR_check.vi"("Driver Name"=w564, "Error Code"=w565, "error in"=w567, "DriverConnect in"=w566) -> ("error out"=w563:T14)  [unwired: 6 in, 1 out]
                }
              }
            }
            frame #2 {
            }
          }
        }
        frame "get" {
          n153 = flat-sequence {
            tunnel: w587 -> [w597]
            tunnel: w588 -> [w598]
            tunnel: w589 -> [w599]
            tunnel: w578 -> [w591]
            tunnel: [w591] -> w586
            tunnel: [w599] -> w585
            tunnel: [w598] -> w584
            tunnel: [w596] -> w583
            tunnel: [w595] -> w582
            tunnel: [w592] -> w581
            tunnel: [w593] -> w580
            tunnel: [w597] -> w579
            tunnel: w577 -> [w594]
            tunnel: w586 -> [w610]
            tunnel: w585 -> [w608]
            tunnel: w584 -> [w607]
            tunnel: w583 -> [w605]
            tunnel: w582 -> [w604]
            tunnel: w581 -> [w603]
            tunnel: w580 -> [w602]
            tunnel: w579 -> [w600]
            tunnel: [w609] -> w576
            tunnel: [w606] -> w575
            tunnel: [w601] -> w574
            tunnel: [w651] -> w590
            tunnel: w576 -> [w651]
            tunnel: w575 -> [w650]
            tunnel: w574 -> [w649]
            tunnel: [w650] -> w573
            tunnel: [w649] -> w572
            frame #0 {
              n154 = Unbundle By Name(w591) -> ("Data.Connect"=w596:T1, "Data.Func"=w595:T7)
              n155 = call "MLLF_CommandDelimeter.vi"("command with param"=w594) -> ("param 1"=w593:string, "command"=w592:string)  [unwired: 6 in, 3 out]
            }
            frame #1 {
              n156 = case shown="\"READ\"" w603 {
                selector: w603 -> [w613 _ _ _]
                tunnel: [w612 w617 w632 w644] -> w606
                tunnel: w608 -> [_ _ _ w643]
                tunnel: [w614 w618 w633 w646] -> w609
                tunnel: w610 -> [w614 w618 w633 w646]
                tunnel: w605 -> [_ _ w625 w645]
                tunnel: w607 -> [_ _ _ w642]
                tunnel: w602 -> [_ _ _ w635]
                tunnel: w604 -> [_ _ _ w641]
                tunnel: ["" w616 w620 w634] -> w601
                tunnel: w600 -> [_ w617 _ _]
                tunnel: [_ _ w619 _] -> _
                frame "False", Default {
                  n157 = call "MLLF_UnknownCommand(SubVI).vi"("Unknown command"=w613) -> ("error out"=w612:errorcluster)  [unwired: 10 in]
                }
                frame "TIMEOUT" {
                  n158 = Unbundle By Name(w618) -> ("Data.Connect.InterfaceSettings.TMO, ms"=w615:i32)
                  n159 = Format Value(value (0)=w615) -> (output string=w616:string)  [unwired: 2 in]
                }
                frame "READ" {
                  n160 = call "MLLF_ClearBuffer.vi"("Timeout(default = 300 ms)"=u32 100, "DriverConnect in"=w625) -> ("Error Out"=w622:errorcluster, "DriverConnect out"=w624:T1, "Cleared"=w619:T17)  [unwired: 6 in]
                  n161 = call "MLLF_WriteToBufferWithDelay.vi"("Delay Time ( 0,05 s)"=0.05 ("Delay Time (s)"), "Command"="READ?" ("String"), "Error In"=w622, "DriverConnect in"=w624) -> ("Error Out"=w631:errorcluster, "DriverConnect out"=w630:T1)  [unwired: 6 in]
                  n162 = call "MLLF_ReadBuffer.vi"("Error In"=w631, "DriverConnect in"=w630) -> ("Error Out"=w632:errorcluster, "String"=w626:string)  [unwired: 6 in, 1 out]
                  n163 = Fract/Exp String To Number(use system decimal point (T)=FALSE, string=w626) -> (number=w621:dbl)  [unwired: 2 in, 1 out]
                  n164 = Format Value(value (0)=w621) -> (output string=w620:string)  [unwired: 2 in]
                }
                frame "SCPI" {
                  n165 = case shown="\"VDC\", Default" w641 {
                    tunnel: [1.0 ("Delay Time (s)") 0.05 ("Delay Time (s)")] -> w636
                    frame "F" {
                    }
                    frame "VDC", Default {
                    }
                  }
                  n166 = call "MLLF_WriteToBufferWithDelay.vi"("Delay Time ( 0,05 s)"=w636, "Command"=w635, "DriverConnect in"=w645) -> ("Error Out"=w640:errorcluster, "DriverConnect out"=w639:T1)  [unwired: 7 in]
                  n167 = call "MLLF_ReadBuffer.vi"("Error In"=w640, "DriverConnect in"=w639) -> ("Error Out"=w638:errorcluster, "DriverConnect out"=w637:T1, "String"=w634:string)  [unwired: 6 in]
                  n168 = call "HP34401A_ESR_check.vi"("Driver Name"=w642, "Error Code"=w643, "error in"=w638, "DriverConnect in"=w637) -> ("error out"=w644:T14)  [unwired: 6 in, 1 out]
                }
              }
            }
            frame #2 {
            }
          }
        }
        frame "close" {
          n169 = Unbundle By Name(w653) -> ("Data.Connect.OpenedSession"=w655:T3)
          n170 = VISA Close(VISA resource name=w655) -> (error out=w654:errorcluster)  [unwired: 1 in]
        }
      }
    }
    frame Error {
    }
  }
  n171 = flat-sequence {
    tunnel: [w667] -> w2
    tunnel: [w666] -> w4
    tunnel: w7 -> [w665]
    tunnel: w5 -> [w664]
    tunnel: w6 -> [w660]
    tunnel: [w662] -> w3
    frame #0 {
      # "driver out"
      n172 = Unbundle By Name(w660) -> ("Data"=w659:cluster{"Connect":T1, "Channel":T6, "Func":T7})
      n173 = To Variant(anything=w659) -> (Variant=w661:variant)
      n174 = Bundle By Name(cluster=w660, "Saved Data"=w661) -> (w662:T8)
      n175 = call "MLLF_SaveLastSettingUtility.vi"("error in"=w664, "Saved Data"=w661) -> ("error out"=w663:T14)  [unwired: 8 in, 1 out]
      n176 = call "MCF_Output.vi"("Error In"=w663, "Input"=w665) -> ("Error Out"=w666:errorcluster, "Output"=w667:string)  [unwired: 8 in]
    }
  }
  n177 = local write "Settings"(w3) -> ()
  "error out" <- w4
  "Response" <- w2
